vi "Filtered Chart (SubVI).vi"(6 "Sample quantity":i32, 9 "Numeric in":i32, 10 "Array in":i32[](array[numeric]), 11 "Numeric 3":i32) -> (1 "Numeric out":i32, 2 "Filtered":i32(graph), 3 "Array out":i32[](array[numeric]))   [LabVIEW 2012]
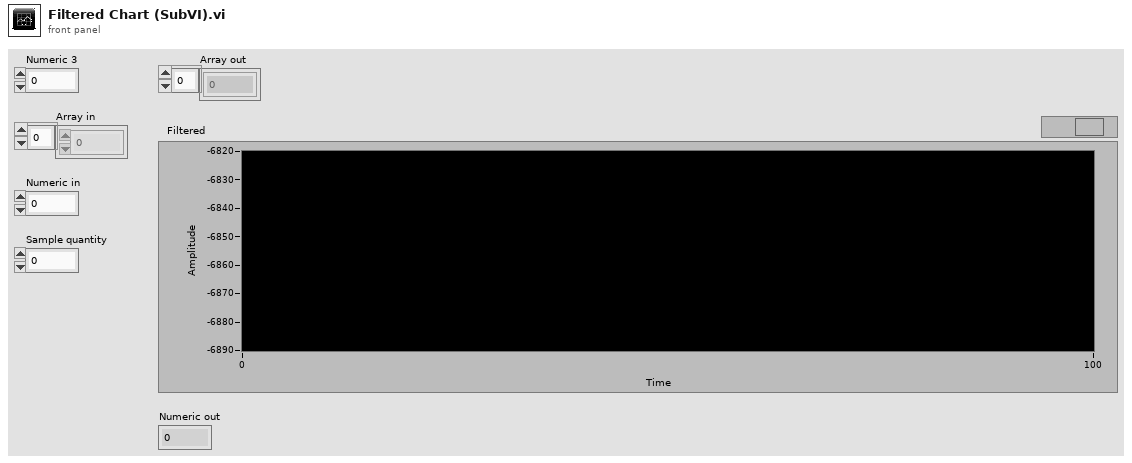
[diagram p1: front panel]
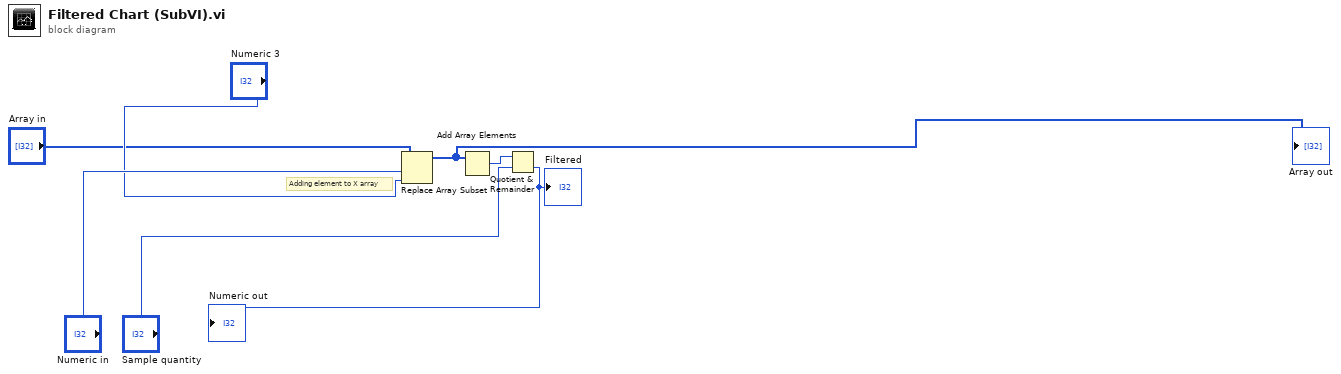
[diagram p0: block diagram]
diagram:
  # "Adding element to X array"
  n1 = Replace Array Subset(array="Array in", new element="Numeric 3", index="Numeric in") -> (w6:i32[])
  "Array out" <- w6
  n2 = Add Array Elements(numeric array=w6) -> (sum=w1:i32)
  n3 = Quotient & Remainder(x=w1, y="Sample quantity") -> (floor(x/y)=→"Filtered" →"Numeric out":i32)  [unwired: 1 out]
